vi "1_0_FFT_conventional representation.vi"() -> ()   [LabVIEW 2009]
uses:
  <vilib>/Analysis/2dsp.llb/Real FFT.vi
  <vilib>/Analysis/NI_AALBase.lvlib
  <vilib>/Analysis/NI_AALPro.lvlib
panel:
  out "Energy":dbl=50.0000000000001
  out "FREQUENCY RESOLUTION":dbl=4.0
  out "?":dbl=200.0
  out "?":string="Nyquist frequency point ="
  out "?":string="+N/2"
  out "?":string="-(N/2-1)"
  out "FFT MAGNITUDE SPECTRUM (conventional representation)":cluster{dbl, "fundamental frequency":dbl, dbl[]}(graph)={-196.0, "fundamental frequency"=4.0, [0.002488126611933955, 0.004827061844930729, 0.006875986932682891, 0.008510386192073796, 0.009629115554022724, 0.010160232942939114, 0.010065276968675952, 0.009341759063947378, 0.008023724973601473, 0.006180339887498948, 0.003912552629743327, 0.0013479931517580627, 0.0013656507965938752, 0.004068452105641516, 0.006596868107423749, 0.008792735013011897, 0.01051217465952634, 0.011633954309217555, 0.012066862159151152, 0.011755705045849463, 0.01068559855063689, 0.00888430033288713, 0.0064224312052753715, 0.003411530727248826, 2.9639425473644758e-18, 0.0036329112344645757, 0.007284818243294948, 0.010739274281135506, 0.013775790643454843, 0.016180339887498948, 0.017755848469349796, 0.018332178605722626, 0.017775116610742287, 0.015993925613800437, 0.012947082651061727, 0.008645900821797406, 0.0031558327897443436, 0.0034046420606902617, 0.010867533000678128, 0.019021130325903073, 0.027617842508120907, 0.03638374936678531, 0.04502946066264226, 0.05326180631376064, 0.060795842914192, 0.06736664342652733, 0.07274034373688162, 0.07672395095836265, 0.07917347255005394, 0.08, 0.07917347255005394, 0.07672395095836265, 0.07274034373688162, 0.06736664342652733, 0.060795842914192, 0.05326180631376064, 0.04502946066264226, 0.03638374936678531, 0.027617842508120907, 0.019021130325903073, 0.010867533000678128, 0.0034046420606902617, 0.0031558327897443436, 0.008645900821797406, 0.012947082651061727, 0.015993925613800437, 0.017775116610742287, 0.018332178605722626, 0.017755848469349796, 0.016180339887498948, 0.013775790643454843, 0.010739274281135506, 0.007284818243294948, 0.0036329112344645757, 2.9639425473644758e-18, 0.003411530727248826, 0.0064224312052753715, 0.00888430033288713, 0.01068559855063689, 0.011755705045849463, 0.012066862159151152, 0.011633954309217555, 0.01051217465952634, 0.008792735013011897, 0.006596868107423749, 0.004068452105641516, 0.0013656507965938752, 0.0013479931517580627, 0.003912552629743327, 0.006180339887498948, 0.008023724973601473, 0.009341759063947378, 0.010065276968675952, 0.010160232942939114, 0.009629115554022724, 0.008510386192073796, 0.006875986932682891, 0.004827061844930729, 0.002488126611933955, 0.0]}
  in  "Deg/Rad":enum16{"Rad", "Deg"}(ring)=enum."Deg"
  in  "Phase Unwrap":bool=TRUE
  in  "Phase correction":bool=TRUE
  out "PHASE SPECTRUM":cluster{dbl, "fundamental frequency":dbl, dbl[]}(graph)={-196.0, "fundamental frequency"=4.0, [77.39999999999998, 64.8, 52.199999999999974, 39.60000000000001, 26.999999999999986, 14.399999999999999, 1.8000000000000245, -10.80000000000005, -23.39999999999998, -35.99999999999999, -48.600000000000044, -61.199999999999974, -73.80000000000003, -86.40000000000003, 81.00000000000004, 68.40000000000002, 55.8, 43.2, 30.60000000000001, 17.999999999999996, 5.3999999999999995, -7.200000000000006, -19.799999999999976, -32.40000000000003, 0.0, -57.59999999999997, -70.19999999999995, -82.8, 84.60000000000001, 72.0, 59.400000000000006, 46.80000000000001, 34.199999999999996, 21.599999999999998, 8.999999999999998, -3.5999999999999632, -16.199999999999896, -28.800000000000026, -41.400000000000034, -54.00000000000001, -66.59999999999998, -79.19999999999999, 88.2, 75.6, 63.000000000000014, 50.39999999999999, 37.800000000000004, 25.199999999999996, 12.600000000000001, 0.0, -12.599999999999971, -25.200000000000024, -37.8, -50.400000000000006, -63.000000000000014, -75.6, -88.2, 79.20000000000002, 66.59999999999998, 54.0, 41.40000000000002, 28.80000000000004, 16.199999999999903, 3.5999999999999814, -9.000000000000007, -21.59999999999998, -34.19999999999999, -46.800000000000004, -59.40000000000001, -71.99999999999999, -84.60000000000004, 82.8, 70.19999999999996, 57.59999999999998, 0.0, 32.4, 19.80000000000001, 7.200000000000006, -5.400000000000005, -18.000000000000014, -30.600000000000026, -43.199999999999996, -55.80000000000001, -68.40000000000002, -81.00000000000003, 86.40000000000002, 73.80000000000004, 61.19999999999993, 48.6, 35.999999999999986, 23.399999999999977, 10.800000000000022, -1.8000000000000416, -14.400000000000013, -26.999999999999986, -39.60000000000004, -52.19999999999997, -64.79999999999998, -77.39999999999999, 0.0]}
  out "TIME DOMAIN WAVEFORM":dbl[](graph)=[1.0, 1.0, 1.0, 1.0, 1.0, 1.0, 1.0, 1.0, 0.0, 0.0, 0.0, 0.0, 0.0, 0.0, 0.0, 0.0, 0.0, 0.0, 0.0, 0.0, 0.0, 0.0, 0.0, 0.0, 0.0, 0.0, 0.0, 0.0, 0.0, 0.0, 0.0, 0.0, 0.0, 0.0, 0.0, 0.0, 0.0, 0.0, 0.0, 0.0, 0.0, 0.0, 0.0, 0.0, 0.0, 0.0, 0.0, 0.0, 0.0, 0.0, 0.0, 0.0, 0.0, 0.0, 0.0, 0.0, 0.0, 0.0, 0.0, 0.0, 0.0, 0.0, 0.0, 0.0, 0.0, 0.0, 0.0, 0.0, 0.0, 0.0, 0.0, 0.0, 0.0, 0.0, 0.0, 0.0, 0.0, 0.0, 0.0, 0.0, 0.0, 0.0, 0.0, 0.0, 0.0, 0.0, 0.0, 0.0, 0.0, 0.0, 0.0, 0.0, 0.0, 0.0, 0.0, 0.0, 0.0, 0.0, 0.0, 0.0]
  in  "stop":bool
  in  "Sampling frequency":i32=400
  in  "# of Samples":i32=100
  in  "SIGNAL TYPE":T1(ring)=enum."PULSE"
  in  "alpha":dbl=0.5
  in  "c":dbl=1.0
  in  "Duty cycle (%)":dbl=50.0 format="%0.2f"
  in  "?":bool=TRUE
  in  "Phase in":dbl format="%0.2f"
  in  "Frequency (f)":dbl=4.0 format="%0.2f"
  in  "Start":dbl format="%0.2f"
  in  "End":dbl=1.0 format="%0.2f"
  in  "Width":i32=8
  in  "Delay":i32
  in  "Amplitude":dbl=1.0 format="%0.2f"
  # "Program Developed by Indranil Sinharoy"
  # "Rad. freq."
  # "Samples"
  # "SAMPLING INFO"
  # "SIGNAL INFORMATION"
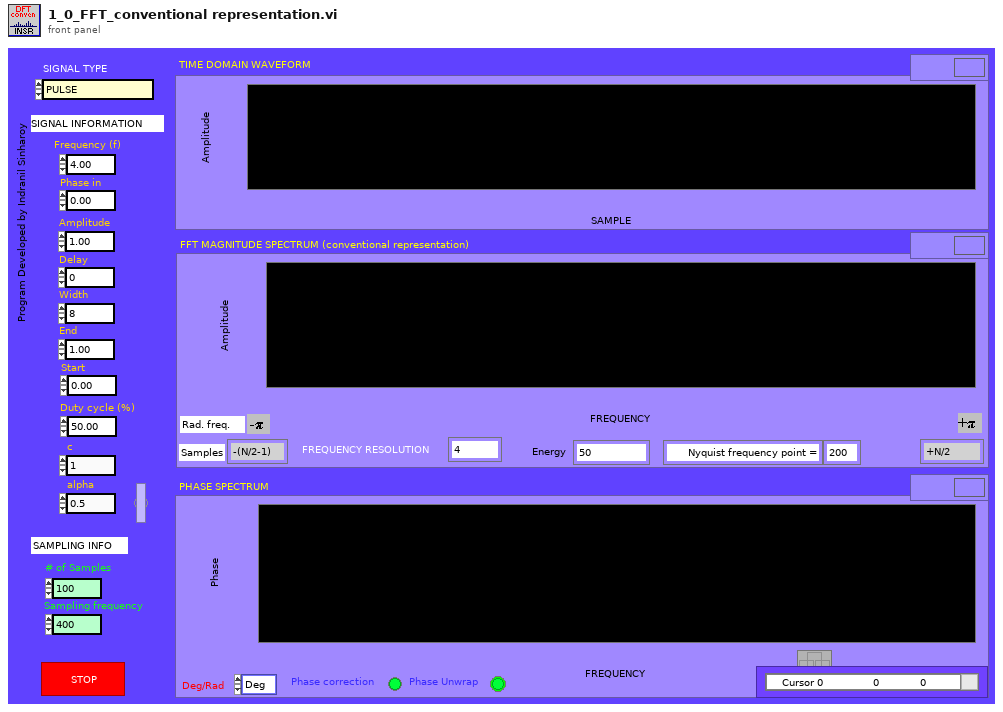
[diagram p1: front panel]
types:
  T1 = enum16{"SINE", "TRIANGLE", "SQUARE", "PULSE", "RAMP", "SAW-TOOTH", "IMPULSE", "REAL EXPONENTIAL"}
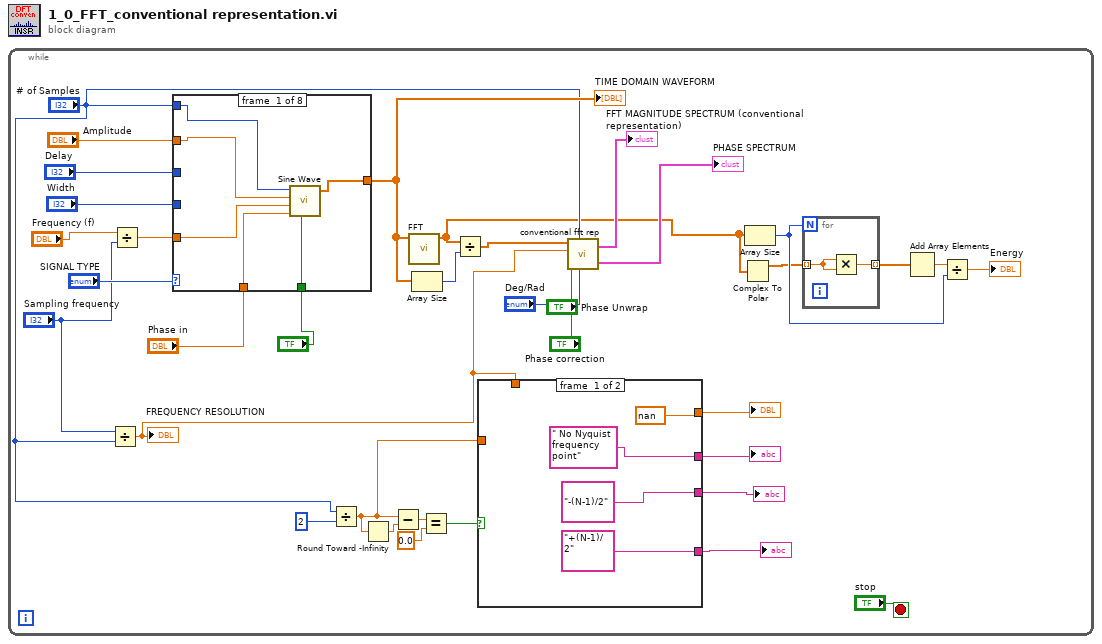
[diagram p0: block diagram]
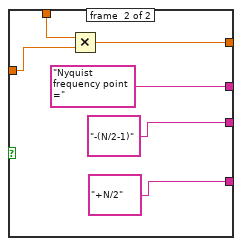
[diagram p2: hidden frame]
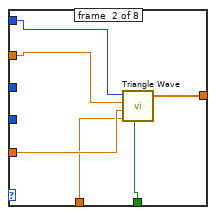
[diagram p3: hidden frame]
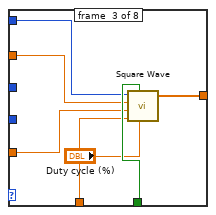
[diagram p4: hidden frame]
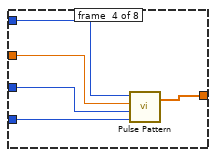
[diagram p5: hidden frame]
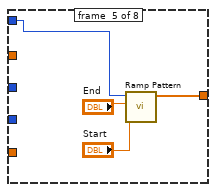
[diagram p6: hidden frame]
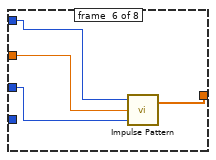
[diagram p7: hidden frame]
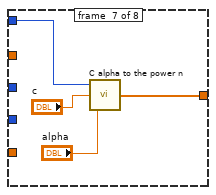
[diagram p8: hidden frame]
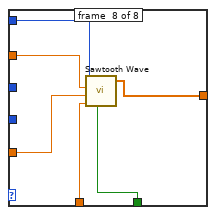
[diagram p9: hidden frame]
diagram:
  n1 = while {
    stop <- "stop" stop-if-true
    n2 = Divide(x="Sampling frequency", y="# of Samples") -> (x/y=w12:dbl)
    "FREQUENCY RESOLUTION" <- w12
    n3 = Divide(x="Frequency (f)", y="Sampling frequency") -> (x/y=w31:dbl)
    n4 = case shown="\"SAW-TOOTH\"" "SIGNAL TYPE" {
      tunnel: "# of Samples" -> [w54 w58 w66 w72 w76 w80 w84 w87]
      tunnel: "Amplitude" -> [w53 w57 w65 w71 _ w79 _ w88]
      tunnel: "Delay" -> [_ _ _ w70 _ w78 _ _]
      tunnel: "Width" -> [_ _ _ w69 _ _ _ _]
      tunnel: [w50 w59 w62 w68 w73 w77 w83 w86] -> w26
      tunnel: w31 -> [w52 w56 w64 _ _ _ _ w89]
      tunnel: "Phase in" -> [w51 w55 w63 _ _ _ _ w90]
      tunnel: "?" -> [w49 w60 w67 _ _ _ _ w85]
      frame #0 {
        n5 = call <vilib>:"Sine Wave.vi"("samples"=w54, "amplitude"=w53, "frequency"=w52, "phase in"=w51, "reset phase"=w49) -> ("sine wave"=w50:dbl[])  [unwired: 2 out]
      }
      frame #1 {
        n6 = call <vilib>:"Triangle Wave.vi"("samples"=w58, "amplitude"=w57, "frequency"=w56, "phase in"=w55, "reset phase"=w60) -> ("triangle wave"=w59:dbl[])  [unwired: 2 out]
      }
      frame #2 {
        n7 = call <vilib>:"Square Wave.vi"("samples"=w66, "reset phase"=w67, "amplitude"=w65, "frequency"=w64, "duty cycle (%)"="Duty cycle (%)", "phase in"=w63) -> ("square wave"=w62:dbl[])  [unwired: 2 out]
      }
      frame #3 {
        n8 = call <vilib>:"Pulse Pattern.vi"("width"=w69, "delay"=w70, "amplitude"=w71, "samples"=w72) -> ("Pulse Pattern"=w68:dbl[])  [unwired: 1 out]
      }
      frame #4 {
        n9 = call <vilib>:"Ramp Pattern.vi"("start"="Start", "end"="End", "samples"=w76) -> ("Ramp Pattern"=w73:dbl[])  [unwired: 7 in, 1 out]
      }
      frame #5 {
        n10 = call <vilib>:"Impulse Pattern.vi"("delay"=w78, "amplitude"=w79, "samples"=w80) -> ("Impulse Pattern"=w77:dbl[])  [unwired: 1 out]
      }
      frame #6 {
        n11 = call "C alpha to the power n.vi"("alpha"="alpha", "c"="c", "n"=w84) -> ("Waveform Graph"=w83:dbl[])
      }
      frame #7 {
        n12 = call <vilib>:"Sawtooth Wave.vi"("samples"=w87, "amplitude"=w88, "frequency"=w89, "phase in"=w90, "reset phase"=w85) -> ("sawtooth wave"=w86:dbl[])  [unwired: 2 out]
      }
    }
    "TIME DOMAIN WAVEFORM" <- w26
    n13 = Divide(x="# of Samples", y=2) -> (x/y=w11:dbl)
    n14 = Round Toward -Infinity(1:w11) -> (0:w20:dbl)
    n15 = Subtract(x=w11, y=w20) -> (x-y=w19:dbl)
    n16 = call-poly <vilib>:"FFT.vi"("X"=w26) -> ("FFT {X}"=w1:cdb[])  [unwired: 9 in, 1 out]
    n17 = Array Size(array=w26) -> (size(s)=w27:i32)
    n18 = Equal?(x=w19, y=0.0) -> (x = y?=w17:bool)
    n19 = Divide(x=w1, y=w27) -> (x/y=w24:cdb[])
    n20 = case shown="False" w17 {
      tunnel: ["-(N-1)/2" "-(N/2-1)"] -> w16
      tunnel: ["+(N-1)/2" "+N/2"] -> w15
      tunnel: [" No Nyquist frequency point" "Nyquist frequency point ="] -> w13
      tunnel: w12 -> [_ w45]
      tunnel: w11 -> [_ w44]
      tunnel: [nan ("y") w43] -> w10
      frame #0 {
      }
      frame #1 {
        n21 = Multiply(x=w45, y=w44) -> (x*y=w43:dbl)
      }
    }
    "?" <- w16
    "?" <- w15
    "?" <- w13
    "?" <- w10
    n22 = call "conventional fft rep.vi"("Deg/Rad"="Deg/Rad", "samples"="# of Samples", "Phase correction"="Phase correction", "Phase Unwrap"="Phase Unwrap", "fundamental frequency"=w12, "fft output"=w24) -> ("Conventional FFT phase"=→"PHASE SPECTRUM":cluster{dbl, "fundamental frequency":dbl, dbl[]}, "Conventional FFT mag"=→"FFT MAGNITUDE SPECTRUM (conventional representation)":cluster{dbl, "fundamental frequency":dbl, dbl[]})
    n23 = Complex To Polar(r * e^(i*theta)=w1) -> (r=w2:dbl[])  [unwired: 1 out]
    n24 = Array Size(array=w1) -> (size(s)=w3:i32)
    n25 = for {
      N: w3 -> [_]
      tunnel: w2 -> [w38] mode=indexing
      tunnel: [w37] -> w6 mode=indexing
      n26 = Multiply(x=w38, y=w38) -> (x*y=w37:dbl)
    }
    n27 = Add Array Elements(numeric array=w6) -> (sum=w5:dbl)
    n28 = Divide(x=w5, y=w3) -> (x/y=→"Energy":dbl)
  }
